vi "MSRV_Concatenate_server_parameters_into_a_string.vi"(0 "Status":bool, 1 "JSON":string, 5 "Data":string, 7 "ErrorStatus":bool, 9 "ErrorCode":i32, 11 "ErrorSourse":string) -> (4 "output JSON":string)   [LabVIEW 2018]
uses:
  <vilib>/addons/Tools/Unicode/UTF8 Tools.lvlib
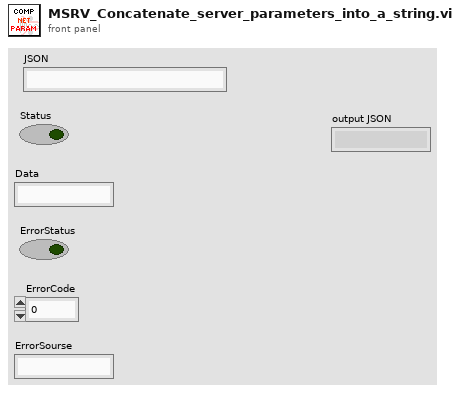
[diagram p1: front panel]
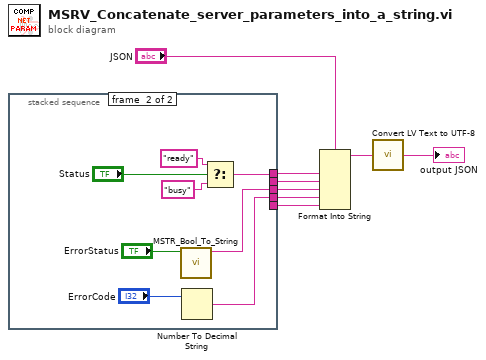
[diagram p0: block diagram]
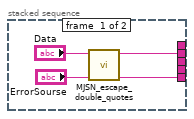
[diagram p2: hidden frame]
diagram:
  n1 = stacked-sequence {
    tunnel: [w11 _] -> w5
    tunnel: [w9 _] -> w4
    tunnel: [_ w19] -> w3
    tunnel: [_ w15] -> w2
    tunnel: [_ w17] -> w1
    frame #0 {
      n2 = call "MJSN_escape_double_quotes.vi"("String in 4"="ErrorSourse", "String in 1"="Data") -> ("String out 4"=w9:string, "String out 1"=w11:string)  [unwired: 6 in, 2 out]
    }
    frame #1 {
      n3 = call "MSTR_Bool_To_String.vi"("Boolean in"="ErrorStatus") -> ("String Boolean out"=w15:string)  [unwired: 10 in]
      n4 = Number To Decimal String(number="ErrorCode") -> (decimal integer string=w17:string)  [unwired: 1 in]
      n5 = Select(t="ready", s="Status", f="busy") -> (s? t:f=w19:string)
    }
  }
  n6 = Format Into String(format string="JSON", w3, w5, w2, w1, w4) -> (resulting string=w7:string)  [unwired: 2 in, 1 out]
  n7 = call <vilib>:"Convert LV Text to UTF-8.vi"("LV Text"=w7) -> ("UTF-8 Text"=→"output JSON":string)  [unwired: 13 in, 1 out]
